vi "Main Engine & TCP Engine Q Init LV2GBL.vi"(6 "Q Option":T1, 8 "error in":errorcluster) -> (0 "error out":errorcluster, 2 "TCP Enigine Tx-Q":refnum<queue>, 3 "Main Engine Tx-Q":refnum<queue>)   [LabVIEW 2024]
doc: "All Rights Reserved © 2023 SyncSols"
uses:
  Controls/Main Engine Q Option.ctl
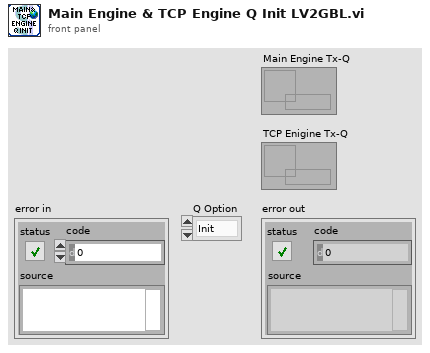
[diagram p1: front panel]
types:
  T1 = typedef "Main Engine Q Option.ctl" = enum16{"Init", "Get"}
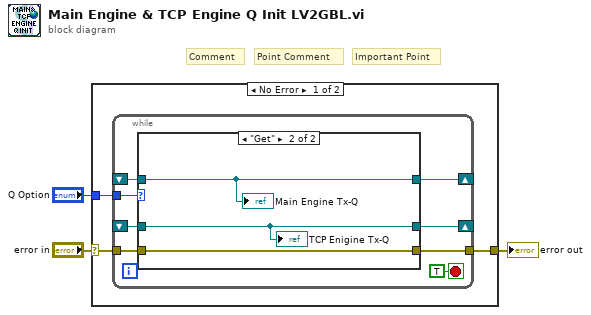
[diagram p0: block diagram]
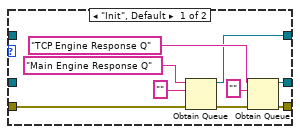
[diagram p2: hidden frame]
diagram:
  # "Important Point"
  # "Point Comment"
  # "Comment"
  n1 = case shown="No Error" "error in" {
    selector: "error in" -> [w6 w27]
    tunnel: [w5 w27] -> w3
    tunnel: "Q Option" -> [w4 _]
    frame No Error {
      n2 = while {
        tunnel: w6 -> [w14]
        tunnel: [w13] -> w5
        tunnel: w4 -> [w10]
        shift-right: [w11] -> _
        shift-left: _ -> [w9]
        shift-right: [w12] -> _
        shift-left: _ -> [w8]
        stop <- TRUE stop-if-true
        n3 = case shown="\"Get\"" w10 {
          tunnel: w14 -> [w18 w26]
          tunnel: [w17 w26] -> w13
          tunnel: [w16 w24] -> w12
          tunnel: [w15 w25] -> w11
          tunnel: w9 -> [_ w25]
          tunnel: w8 -> [_ w24]
          frame "Init", Default {
            n4 = Obtain Queue(name (unnamed)="Main Engine Response Q", element data type="", error in (no error)=w18) -> (queue out=w15:refnum<queue>, error out=w21:errorcluster)  [unwired: 2 in, 1 out]
            n5 = Obtain Queue(name (unnamed)="TCP Engine Response Q", element data type="", error in (no error)=w21) -> (queue out=w16:refnum<queue>, error out=w17:errorcluster)  [unwired: 2 in, 1 out]
          }
          frame "Get" {
            "Main Engine Tx-Q" <- w25
            "TCP Enigine Tx-Q" <- w24
          }
        }
      }
    }
    frame Error {
    }
  }
  "error out" <- w3
